vi "SIOSIfmStop.vi"(1 "deviceNumber":i32) -> (0 "success":i32)   [LabVIEW 2009]
uses:
  siosifm.dll
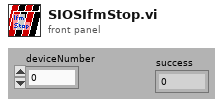
[diagram p1: front panel]
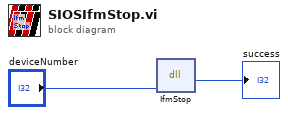
[diagram p0: block diagram]
diagram:
  n1 = dll-call lib="D:/Support/Labview/RE-10/SIOS_IfmDLL/siosifm.dll" fn="IfmStop"("deviceNumber"="deviceNumber") -> ("success"=→"success":i32)  [unwired: 4 in, 2 out]
